vi "correct depth etc.vi"(0 "Correct Depth":dbl format="%.2f", 1 "Incorrect Depth":dbl format="%.2f", 2 "First Absolute Depth":sgl format="%.2f", 3 "Uncorrected Array":dbl[][](array[numeric]) format="%.2f", 4 "New Stainless Feet":i32) -> (5 "Corrected Array":dbl[][](array[numeric]) format="%.5f")   [LabVIEW 2016]
uses:
  Kpro Globals.vi
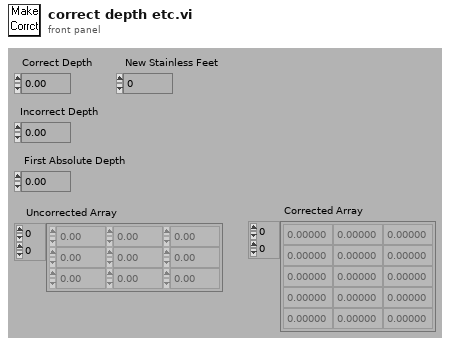
[diagram p1: front panel]
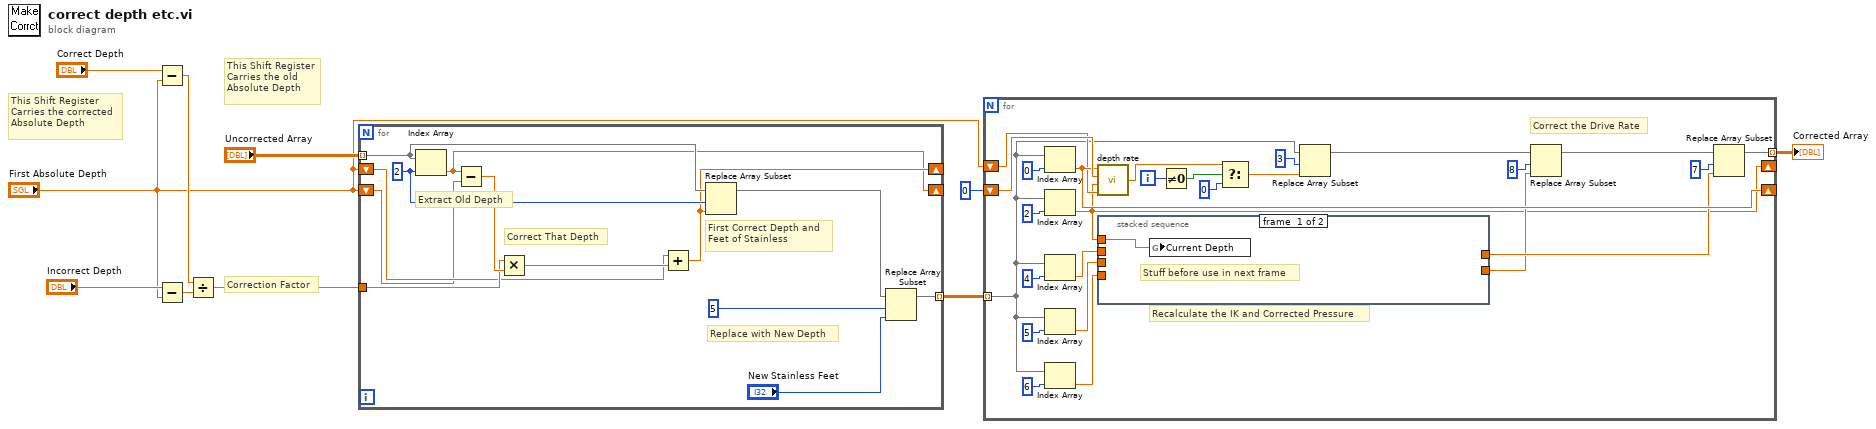
[diagram p0: block diagram]
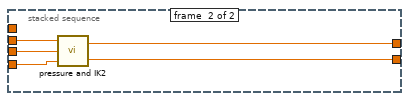
[diagram p2: hidden frame]
diagram:
  # "This Shift Register\nCarries the old\nAbsolute Depth"
  # "This Shift Register\nCarries the corrected \nAbsolute Depth"
  # "Correction Factor"
  n1 = Subtract(x="Correct Depth", y="First Absolute Depth") -> (x-y=w5:dbl)
  n2 = Subtract(x="Incorrect Depth", y="First Absolute Depth") -> (x-y=w3:dbl)
  n3 = Divide(x=w5, y=w3) -> (x/y=w1:dbl)
  n4 = for {
    tunnel: "Uncorrected Array" -> [w22] mode=indexing
    shift-right: [w18] -> _
    shift-left: "First Absolute Depth" -> [w16]
    tunnel: [w14] -> w8 mode=indexing
    tunnel: w1 -> [w20]
    shift-right: [w17] -> _
    shift-left: "First Absolute Depth" -> [w15]
    w23 = 2
    # "Replace with New Depth"
    # "Correct That Depth"
    # "Extract Old Depth"
    # "First Correct Depth and \nFeet of Stainless"
    n5 = Index Array(array=w22, index=w23) -> (element=w17:dbl)
    n6 = Subtract(x=w17, y=w15) -> (x-y=w21:dbl)
    n7 = Multiply(x=w20, y=w21) -> (x*y=w19:dbl)
    n8 = Add(x=w16, y=w19) -> (x+y=w18:dbl)
    n9 = Replace Array Subset(array=w22, new element=w18, index=w23) -> (w13:dbl[])
    n10 = Replace Array Subset(array=w13, new element="New Stainless Feet", index=5) -> (w14:dbl[])
  }
  n11 = for {
    tunnel: w8 -> [w31] mode=indexing
    shift-right: [w24] -> _
    shift-left: "First Absolute Depth" -> [w39]
    shift-right: [w43] -> _
    shift-left: 0 -> [w44]
    tunnel: [w36] -> w6 mode=indexing
    i -> [w49]
    # "Recalculate the IK and Corrected Pressure"
    # "Correct the Drive Rate"
    n12 = Index Array(array=w31, index=0) -> (element=w43:dbl)
    n13 = Index Array(array=w31, index=2) -> (element=w24:dbl)
    n14 = Index Array(array=w31, index=4) -> (element=w30:dbl)
    n15 = Index Array(array=w31, index=5) -> (element=w29:dbl)
    n16 = Index Array(array=w31, index=6) -> (element=w28:dbl)
    n17 = call "depth rate.vi"("Depth Last"=w39, "Depth Current"=w24, "Time Last"=w44, "Time Current"=w43) -> ("Depth Rate"=w46:dbl)
    n18 = stacked-sequence {
      tunnel: [_ w55] -> w35
      tunnel: [_ w54] -> w34
      tunnel: w30 -> [_ w53]
      tunnel: w29 -> [_ w52]
      tunnel: w28 -> [_ w51]
      tunnel: w24 -> [w50 _]
      frame #0 {
        # "Stuff before use in next frame"
        n19 = global write "Kpro Globals.vi" "Current Depth"(w50) -> ()
      }
      frame #1 {
        n20 = call "pressure and IK2.vi"("Pressure"=w51, "Ft. of SS"=w52, "flow"=w53) -> ("Corrected Headloss"=w54:dbl, "IK"=w55:dbl)
      }
    }
    n21 = Not Equal To 0?(x=w49) -> (x != 0?=w48:bool)
    n22 = Select(t=w46, s=w48, f=0) -> (s? t:f=w45:dbl)
    n23 = Replace Array Subset(array=w31, new element=w45, index=3) -> (w38:dbl[])
    n24 = Replace Array Subset(array=w38, new element=w34, index=8) -> (w37:dbl[])
    n25 = Replace Array Subset(array=w37, new element=w35, index=7) -> (w36:dbl[])
  }
  "Corrected Array" <- w6
